vi "CalculateMenuItemIndex.vi"(8 "error in (no error)":errorcluster, 10 "position":cluster{"left":u32, "top":u32}, 11 "menu in":refnum<class "menu.lvclass">) -> (0 "error out":errorcluster, 2 "menu item index":i32, 3 "menu out":refnum<class "menu.lvclass">)   [LabVIEW 2009, in "menu.lvclass"]
uses:
  menu.lvclass
  menu.lvclass/menu.ctl
  Menu Item/menu item.lvclass
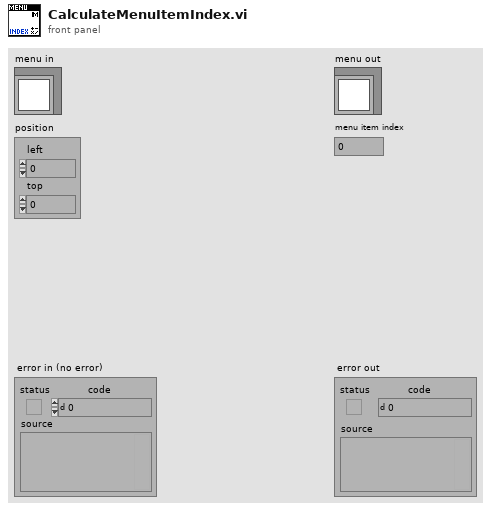
[diagram p1: front panel]
types:
  T1 = cluster{"left":i16, "top":i16, "right":i16, "bottom":i16}
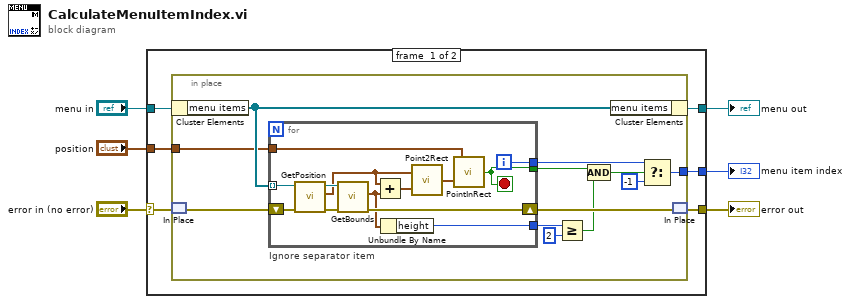
[diagram p0: block diagram]
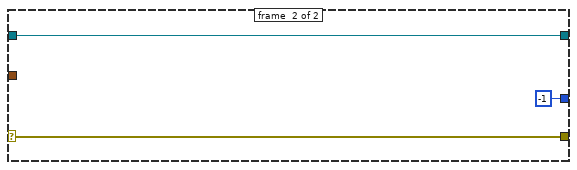
[diagram p2: hidden frame]
diagram:
  n1 = case shown="No Error" "error in (no error)" {
    selector: "error in (no error)" -> [w8 w40]
    tunnel: [w9 w40] -> w3
    tunnel: [w11 w39] -> w5
    tunnel: "menu in" -> [w12 w39]
    tunnel: "position" -> [w10 _]
    tunnel: [w7 -1 ("f")] -> w1
    frame #0 {
      n2 = in-place {
        in-place-border: w10 -> [w23]
        in-place-border: [w18] -> w7
        n3 = in-place-cluster #1(w12) -> ("menu items"=w24:refnum<class "menu item.lvclass">[])
        n4 = in-place-match #2(w8) -> (w22:errorcluster)
        n5 = for "Ignore separator item" {
          tunnel: w24 -> [w37] mode=indexing
          tunnel: [w31] -> w15
          tunnel: [w30] -> w20
          shift-right: [w28] -> w21
          shift-left: w22 -> [w29]
          tunnel: w23 -> [w27]
          tunnel: [w25] -> w17
          i -> [w30]
          stop <- w31 stop-if-true
          n6 = call-dynamic "GetPosition.vi"("error in (no error)"=w29, "menu item in"=w37) -> ("error out"=w35:errorcluster, "position"=w33:cluster{"left":u32, "top":u32}, "menu item out"=w36:refnum<class "menu item.lvclass">)  [unwired: 7 in]
          n7 = call-dynamic "GetBounds.vi"("error in (no error)"=w35, "menu item in"=w36) -> ("error out"=w28:errorcluster, "bounds"=w26:cluster{"width":u32, "height":u32})  [unwired: 7 in, 1 out]
          n8 = Add(x=w33, y=w26) -> (x+y=w34:cluster{u32, u32})
          n9 = Unbundle By Name(w26) -> ("height"=w25:u32)
          n10 = call <vilib>:"Point2Rect.vi"("point b"=w34, "point a"=w33) -> ("rect"=w32:T1)
          n11 = call <vilib>:"PointInRect.vi"("rect"=w32, "point"=w27) -> ("pt in rect"=w31:bool)
        }
        n12 = Greater Or Equal?(x=w17, y=u32 2) -> (x >= y?=w13:bool)
        n13 = Compound Arithmetic op=AND(w15, w13) -> (w14:bool)
        n14 = in-place-cluster #1("menu items"=w24) -> (w11:refnum<class "menu.lvclass">)
        n15 = Select(t=w20, s=w14, f=-1) -> (s? t:f=w18:i32)
        n16 = in-place-match #2(w21) -> (w9:errorcluster)
      }
    }
    frame #1 {
    }
  }
  "menu out" <- w5
  "error out" <- w3
  "menu item index" <- w1
